vi "Compute DistanceToCones.vi"(6 "Target Width (in)":dbl=6.0 format="%#_13g", 8 "results":T1, 10 "FOV":dbl=41.0, 11 "Image Src":T2) -> (0 "results out":T1, 1 "Off Angle":dbl, 3 "Image Dst Out":T2)   [LabVIEW 2025]
doc: "Using the camera lens information and the real world size of the target, use trig and ratios to determine the distance to the target. Also returns the location relative to the image center in a (-1 , 1) coordinate system that may be useful for steering the robot."
uses:
  <vilib>/vision/Image Controls.llb/IMAQ Image.ctl
  Target Fields.ctl
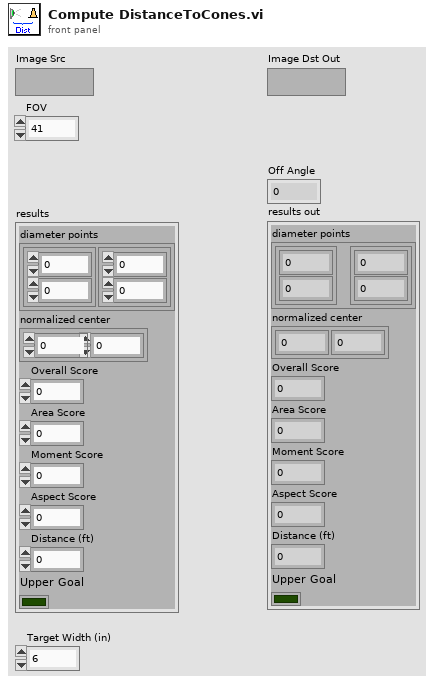
[diagram p1: front panel]
types:
  T1 = typedef "Target Fields.ctl" = cluster{"diameter points":cluster{"first point":cluster{"x":dbl, "y":dbl}, "projected point":cluster{"x":dbl, "y":dbl}}, "normalized center":cluster{"x":dbl, "y":dbl}, "Overall Score":dbl, "Area Score":dbl, "Moment Score":dbl, "Aspect Score":dbl, "Distance (ft)":dbl, "Upper Goal":bool}
  T2 = typedef "IMAQ Image.ctl" = refnum<image>
  T3 = cluster{"first point":cluster{"x":dbl, "y":dbl}, "projected point":cluster{"x":dbl, "y":dbl}}
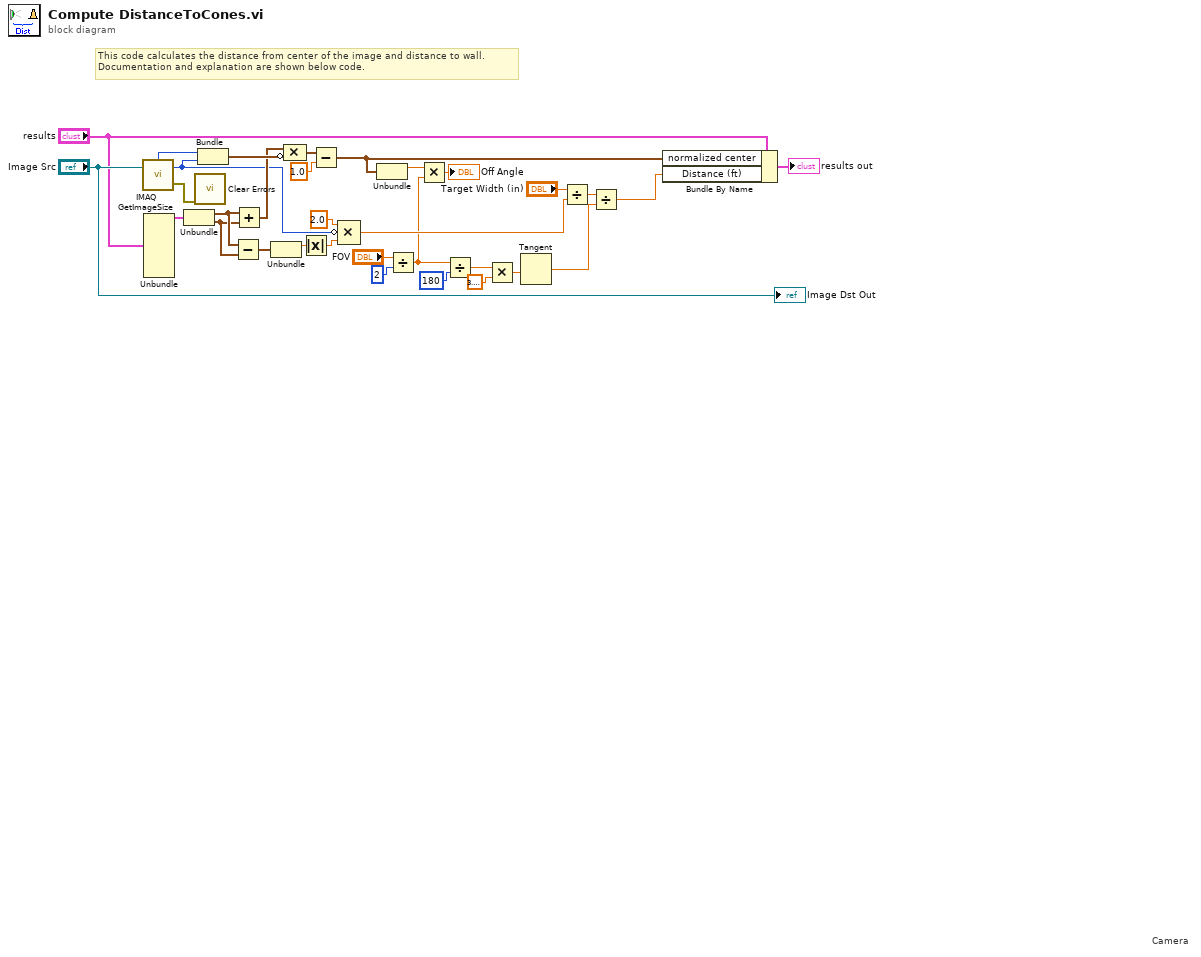
[diagram p0: block diagram]
diagram:
  # "Camera"
  # "This code calculates the distance from center of the image and distance to wall.\nDocumentation and explanation are shown below code."
  n1 = call "IMAQ GetImageSize"("Image"="Image Src") -> ("Y Resolution"=w10:i32, "X Resolution"=w7:i32, "error out"=w24:errorcluster)  [unwired: 3 in]
  n2 = Unbundle("results") -> ("diameter points"=w17:T3)  [unwired: 7 out]
  n3 = Unbundle(w17) -> ("first point"=w14:cluster{"x":dbl, "y":dbl}, "projected point"=w13:cluster{"x":dbl, "y":dbl})
  n4 = call <vilib>:"Clear Errors.vi"("error in (no error)"=w24) -> ()  [unwired: 5 in, 2 out]
  n5 = Bundle("X Resolution"=w7, "Y Resolution"=w10) -> (w15:cluster{"X Resolution":i32, "Y Resolution":i32})  [unwired: 1 in]
  n6 = Subtract(x=w14, y=w13) -> (x-y=w21:cluster{"x":dbl, "y":dbl})
  n7 = Add(x=w14, y=w13) -> (x+y=w12:cluster{"x":dbl, "y":dbl})
  n8 = Unbundle(w21) -> ("x"=w20:dbl)  [unwired: 1 out]
  n9 = Compound Arithmetic op=MULTIPLY(w12, invert w15) -> (w16:cluster{dbl, dbl})
  n10 = Absolute Value(x=w20) -> (abs(x)=w22:dbl)
  n11 = Subtract(x=w16, y=1.0) -> (x-y=w8:cluster{dbl, dbl})
  n12 = Compound Arithmetic op=MULTIPLY(2.0, invert w10, w22) -> (w25:dbl)
  n13 = Unbundle(w8) -> (w5:dbl)  [unwired: 1 out]
  n14 = Divide(x="FOV", y=2) -> (x/y=w2:dbl)
  n15 = Multiply(x=w5, y=w2) -> (x*y=→"Off Angle":dbl)
  n16 = Divide(x=w2, y=180) -> (x/y=w29:dbl)
  n17 = Multiply(x=w29, y=3.141592653589793) -> (x*y=w30:dbl)
  n18 = Tangent(1:w30) -> (0:w27:dbl)
  n19 = Divide(x="Target Width (in)", y=w25) -> (x/y=w4:dbl)
  n20 = Divide(x=w4, y=w27) -> (x/y=w1:dbl)
  n21 = Bundle By Name(cluster="results", "normalized center"=w8, "Distance (ft)"=w1) -> (→"results out":T1)
  "Image Dst Out" <- "Image Src"
